vi "main004_EPICS.vi"() -> ()   [LabVIEW 2020]
uses:
  <vilib>/DAQmx/write.llb/DAQmx Write (Analog DBL 1Chan 1Samp).vi
  <vilib>/DAQmx/miscellaneous.llb/DAQmx Fill In Error Info.vi
  <vilib>/DAQmx/create/channels.llb/DAQmx Create Channel (AO-Voltage-Basic).vi
  <userlib>/caLab/Private/Put_DBL_PV.vi
  libs/Newport ESP301/Newport ESP301.lvlib
panel:
  in  "Path file to softIOC.dbd":string="C:\\Program Files (x86)\\National Instruments\\LabVIEW 2015\\user.lib\\caLab\\lib"
  out "IOC started":bool=TRUE
  in  "Config File":path=path "T:/trARPES/Labview/Front ends/METIS_delayscan/delayScanEPICS.conf" caption="Soft IOC configuration file"
  in  "Configuration Set":T1(array[cluster])=[{"PV name"="trARPES:DelayStage:t0", "description"="Delay Stage time zero Position", "data type"="ai", "number of elements (waveform only)"=1, "element size (waveform only)"="", []}, {"PV name"="trARPES:DelayStage:p1", "description"="Delay Stage range start", "data type"="ai", "number of elements (waveform only)"=1, "element size (waveform only)"="", []}, {"PV name"="trARPES:DelayStage:p2", "description"="Delay Stage range end", "data type"="ai", "number of elements (waveform only)"=1, "element size (waveform only)"="", []}, {"PV name"="trARPES:DelayStage:Pos", "description"="Current Delay Stage position", "data type"="ai", "number of elements (waveform only)"=1, "element size (waveform only)"="", []}]
  in  "Boolean":bool
  out "a":waveform(dbl)(graph)={"t0"=timestamp(3671595662.0560446 s since 1904-01-01), "dt"=1.0, "Y"=[-30.78165]}
  out "Waveform Chart":dbl(graph)=5.25341140860948
  out "x*y":dbl=-1720.2895668242609
  in  "physical channels":tag="Dev1/ao1"
  out "DAC error":errorcluster
  out "ESP error":errorcluster
  out "run?":bool
  in  "set_vel":bool
  in  "velocity [fs/s]":dbl=66.71281903963042
  in  "vel_mm":dbl=0.2 caption="velocity [mm/s]"
  out "meas. velocity":dbl
  in  "stop":bool
  out "output voltage":dbl
  in  "start":bool
  in  "go2p1":bool
  out "position [fs]":dbl=-215785.61526054132
  out "position [mm]":dbl=-30.78165
  in  "p2 [mm]":dbl=1.6200981145
  in  "p1 [mm]":dbl=1.4702018855
  in  "interpolate output":bool
  in  "t2 [fs]":dbl=375.58059249108845
  in  "t1 [fs]":dbl=-624.4194075089106
  in  "t0 [mm]":dbl=1.5638
  in  "Axis (1)":i32=3 min=1 max=3
  in  "Serial Link (RS232)":enum16{"RS232", "USB"}(ring)
  in  "VISA resource name":refnum<visa-resource-name>="COM8"
  in  "main_close":bool=TRUE
  # "Always use CLOSE button to correctly disconnect the device. STOP program afterwards."
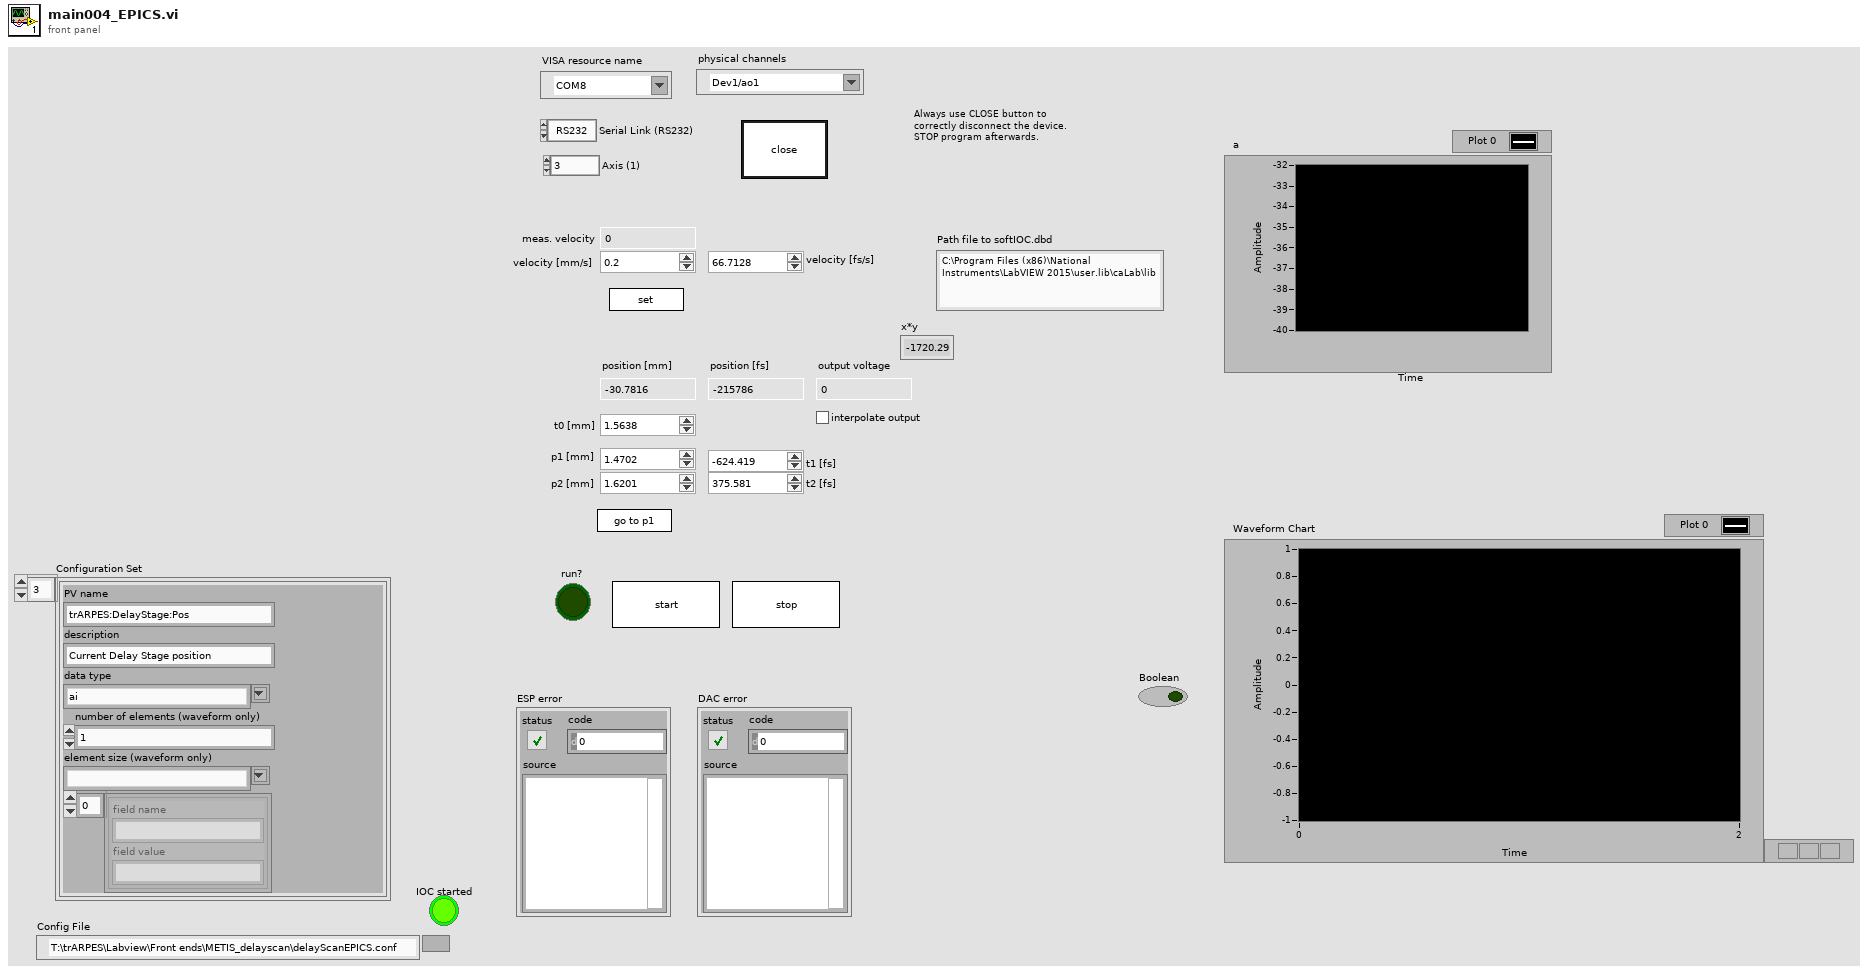
[diagram p1: front panel]
types:
  T1 = cluster{"PV name":string, "description":string, "data type":string, "number of elements (waveform only)":i32, "element size (waveform only)":string, cluster{"field name":string, "field value":string}[]}[]
  T2 = cluster{"dev1_data":refnum<queue>, "dev2_data":refnum<queue>}
  T3 = cluster{"dev1_cmd":refnum<queue>, "dev2_cmd":refnum<queue>}
  T4 = cluster{"PV Name":string, "Data Type":string, "Fields":cluster{"Field Name":string, "Field Value":string}[]}[]
  T5 = cluster{"PV Name":string, "Data Type":string, "Fields":cluster{"Field Name":string, "Field Value":string}[]}
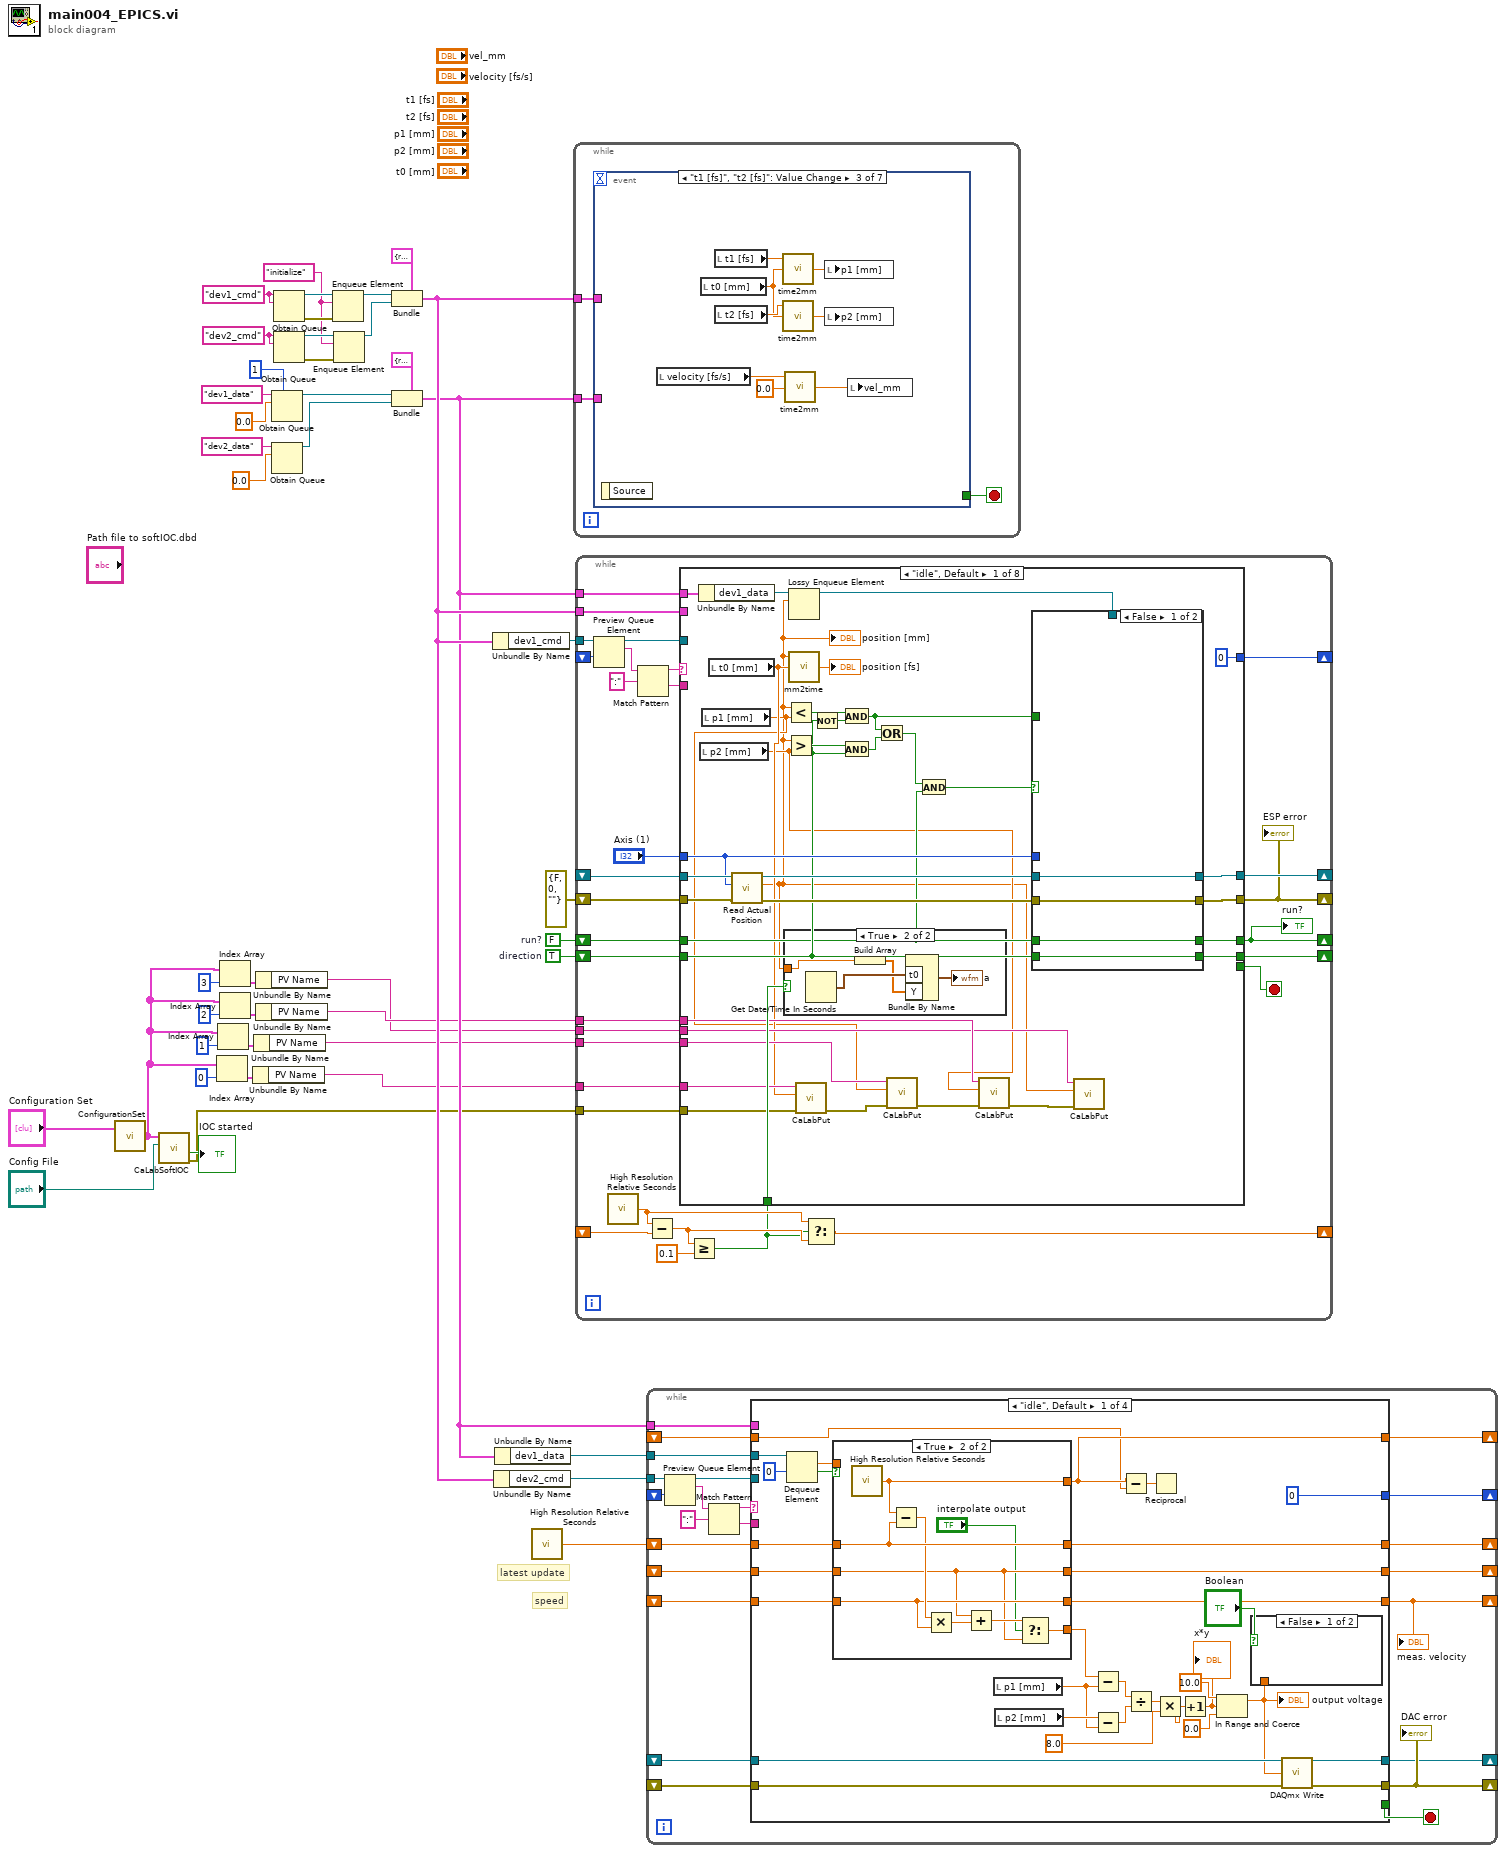
[diagram p0: block diagram]
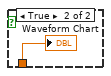
[diagram p2: hidden frame]
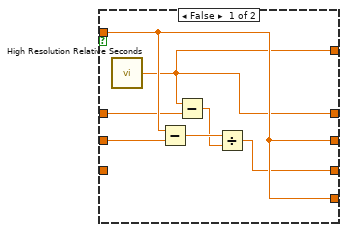
[diagram p3: hidden frame]
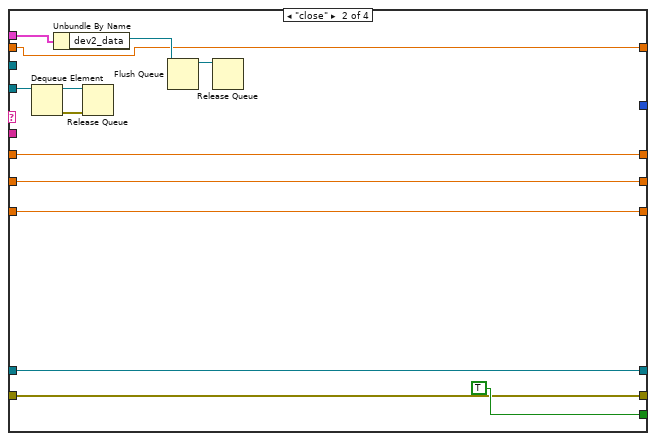
[diagram p4: hidden frame]
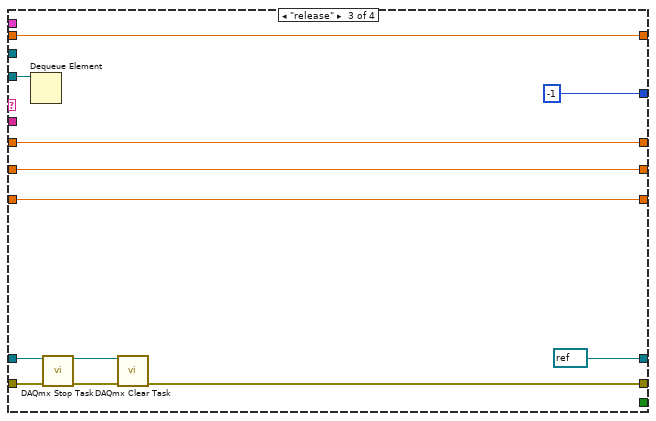
[diagram p5: hidden frame]
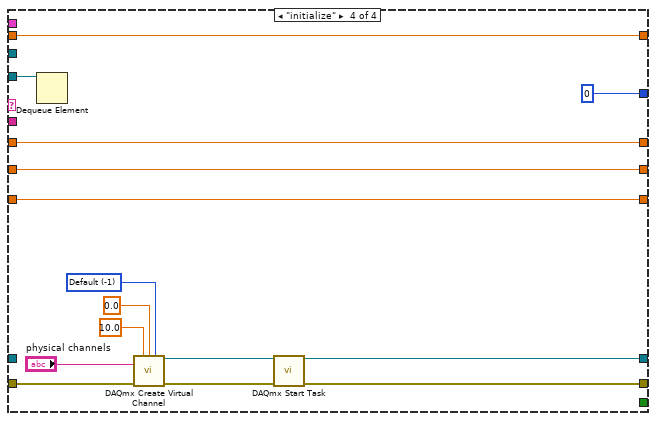
[diagram p6: hidden frame]
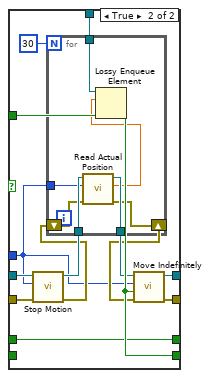
[diagram p8: hidden frame]
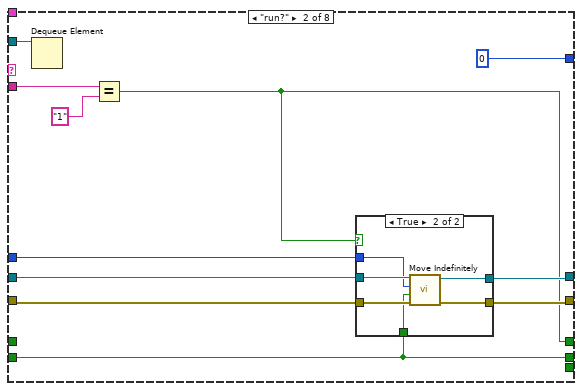
[diagram p9: hidden frame]
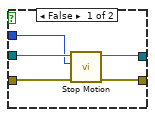
[diagram p10: hidden frame]
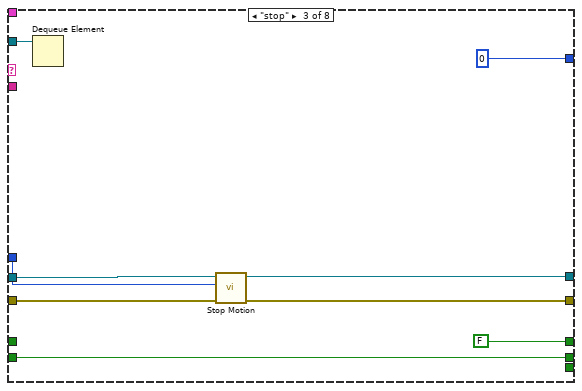
[diagram p11: hidden frame]
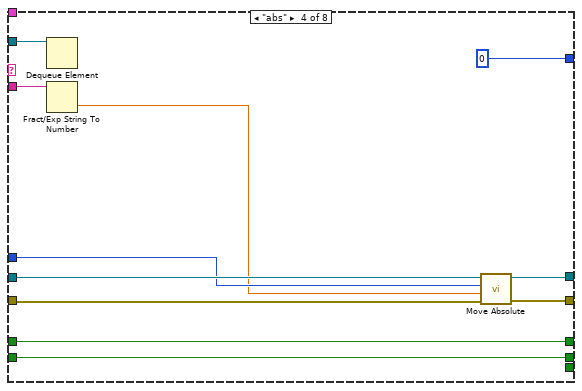
[diagram p12: hidden frame]
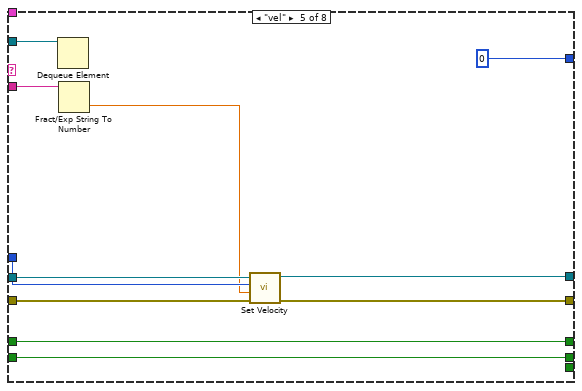
[diagram p13: hidden frame]
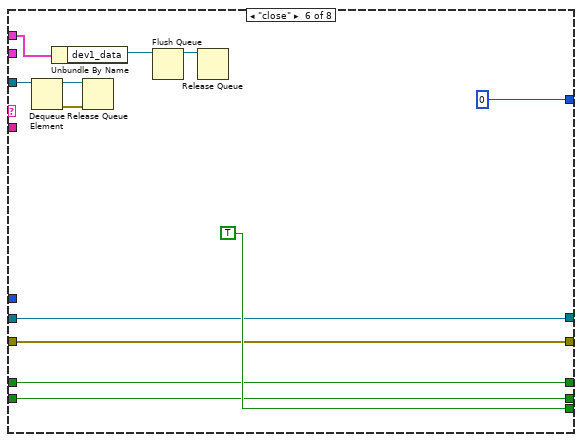
[diagram p14: hidden frame]
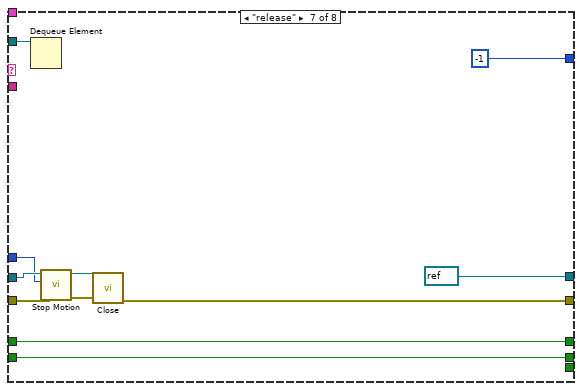
[diagram p15: hidden frame]
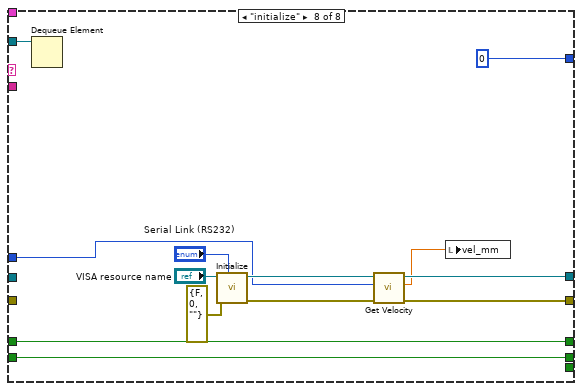
[diagram p16: hidden frame]
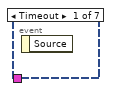
[diagram p17: hidden frame]
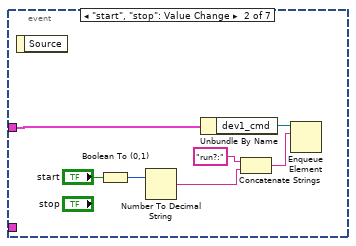
[diagram p18: hidden frame]
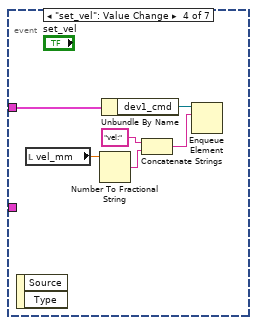
[diagram p19: hidden frame]
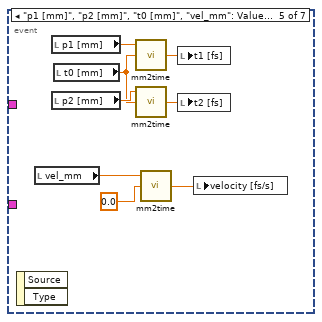
[diagram p20: hidden frame]
diagram:
  w18 = TRUE  # direction
  w21 = FALSE  # run?
  w32 = "dev2_cmd" ("name (unnamed)")
  w38 = "initialize" ("element")
  w33 = "dev1_cmd" ("name (unnamed)")
  # "speed"
  # "latest update"
  n1 = call <userlib>:"ConfigurationSet.vi"("Configuration Set"="Configuration Set") -> ("PV set"=w5:T4)  [unwired: 1 in]
  n2 = call <userlib>:"CaLabSoftIOC.vi"("Config File"="Config File", "PV set"=w5) -> ("error out"=w13:errorcluster, "IOC started"=→"IOC started":bool)  [unwired: 4 in, 2 out]
  n3 = Index Array(array=w5, index=0) -> (element=w16:T5)
  n4 = Index Array(array=w5, index=1) -> (element=w10:T5)
  n5 = Index Array(array=w5, index=3) -> (element=w6:T5)
  n6 = Index Array(array=w5, index=2) -> (element=w9:T5)
  n7 = Unbundle By Name(w16) -> ("PV Name"=w12:string)
  n8 = Unbundle By Name(w10) -> ("PV Name"=w4:string)
  n9 = Unbundle By Name(w6) -> ("PV Name"=w2:string)
  n10 = Unbundle By Name(w9) -> ("PV Name"=w3:string)
  n11 = Obtain Queue(max queue size (-1, unlimited)=1, name (unnamed)="dev1_data", element data type=0.0) -> (queue out=w29:refnum<queue>)  [unwired: 2 in, 2 out]
  n12 = Obtain Queue(name (unnamed)="dev2_data", element data type=0.0) -> (queue out=w28:refnum<queue>)  [unwired: 3 in, 2 out]
  n13 = Obtain Queue(name (unnamed)=w33, element data type=w33) -> (queue out=w44:refnum<queue>, error out=w43:errorcluster)  [unwired: 3 in, 1 out]
  n14 = Obtain Queue(name (unnamed)=w32, element data type=w32) -> (queue out=w39:refnum<queue>, error out=w40:errorcluster)  [unwired: 3 in, 1 out]
  n15 = Enqueue Element(queue=w44, element=w38, error in (no error)=w43) -> (queue out=w41:refnum<queue>)  [unwired: 1 in, 2 out]
  n16 = Enqueue Element(queue=w39, element=w38, error in (no error)=w40) -> (queue out=w37:refnum<queue>)  [unwired: 1 in, 2 out]
  n17 = Bundle(cluster=T3 {"dev1_cmd"=refnum, "dev2_cmd"=refnum}, "dev1_cmd"=w41, "dev2_cmd"=w37) -> (w25:T3)
  n18 = Bundle(cluster=T2 {"dev1_data"=refnum, "dev2_data"=refnum}, "dev1_data"=w29, "dev2_data"=w28) -> (w19:T2)
  n19 = Unbundle By Name(w25) -> ("dev1_cmd"=w34:refnum<queue>)
  n20 = Unbundle By Name(w25) -> ("dev2_cmd"=w24:refnum<queue>)
  n21 = Unbundle By Name(w19) -> ("dev1_data"=w23:refnum<queue>)
  n22 = call <vilib>:"High Resolution Relative Seconds.vi"() -> ("relative seconds"=w22:dbl)
  n23 = while {
    tunnel: w25 -> [w47]
    tunnel: w19 -> [w46]
    stop <- w45 stop-if-true
    n24 = event shown="[2] \"t1 [fs]\", \"t2 [fs]\": Value Change" {
      selector: _ -> [_ _ _ _ _ _ _]
      dyn-events: _ -> [_ _ _ _ _ _ _]
      timeout: _ -> [_ _ _ _ _ _ _]
      tunnel: w47 -> [_ w51 _ w64 _ w82 w85]
      tunnel: w46 -> [_ _ _ _ _ _ _]
      tunnel: [_ _ _ _ _ _ TRUE] -> w45
      event Timeout {
        n25 = event-data() -> ()  [unwired: 1 in, 1 out]
      }
      event "start", "stop": Value Change {
        n26 = event-data() -> ()  [unwired: 1 in, 1 out]
        n27 = Boolean To (0,1)(Boolean="start") -> (0, 1=w49:i16)
        n28 = Number To Decimal String(number=w49) -> (decimal integer string=w48:string)  [unwired: 1 in]
        n29 = Unbundle By Name(w51) -> ("dev1_cmd"=w54:refnum<queue>)
        n30 = Concatenate Strings("run?:" ("string"), w48) -> (w53:string)
        n31 = Enqueue Element(queue=w54, element=w53) -> ()  [unwired: 2 in, 3 out]
      }
      event "t1 [fs]", "t2 [fs]": Value Change {
        n32 = event-data() -> ()  [unwired: 1 in, 1 out]
        n33 = local read "velocity [fs/s]"() -> (w57:dbl)
        n34 = local read "t0 [mm]"() -> (w60:dbl)
        n35 = local read "t1 [fs]"() -> (w61:dbl)
        n36 = local read "t2 [fs]"() -> (w62:dbl)
        n37 = call "time2mm.vi"("Offset (mm)"=w60, "time"=w61) -> ("position (mm)"=w58:dbl)  [unwired: 1 in]
        n38 = call "time2mm.vi"("Offset (mm)"=w60, "time"=w62) -> ("position (mm)"=w59:dbl)  [unwired: 1 in]
        n39 = call "time2mm.vi"("Offset (mm)"=0.0, "time"=w57) -> ("position (mm)"=w55:dbl)  [unwired: 1 in]
        n40 = local write "p1 [mm]"(w58) -> ()
        n41 = local write "p2 [mm]"(w59) -> ()
        n42 = local write "vel_mm"(w55) -> ()
      }
      event "set_vel": Value Change {
        n43 = event-data() -> ()  [unwired: 1 in, 2 out]
        n44 = local read "vel_mm"() -> (w63:dbl)
        n45 = Number To Fractional String(number=w63) -> (F-format string=w67:string)  [unwired: 3 in]
        n46 = Unbundle By Name(w64) -> ("dev1_cmd"=w68:refnum<queue>)
        n47 = Concatenate Strings("vel:" ("string"), w67) -> (w66:string)
        n48 = Enqueue Element(queue=w68, element=w66) -> ()  [unwired: 2 in, 3 out]
      }
      event "p1 [mm]", "p2 [mm]", "t0 [mm]", "vel_mm": Value Change {
        n49 = event-data() -> ()  [unwired: 1 in, 2 out]
        n50 = local read "vel_mm"() -> (w71:dbl)
        n51 = local read "p1 [mm]"() -> (w75:dbl)
        n52 = local read "p2 [mm]"() -> (w76:dbl)
        n53 = local read "t0 [mm]"() -> (w74:dbl)
        n54 = call "mm2time.vi"("Offset (mm)"=w74, "distance (mm)"=w75) -> ("time in fs"=w72:dbl)  [unwired: 1 in]
        n55 = call "mm2time.vi"("Offset (mm)"=w74, "distance (mm)"=w76) -> ("time in fs"=w73:dbl)  [unwired: 1 in]
        n56 = call "mm2time.vi"("Offset (mm)"=0.0, "distance (mm)"=w71) -> ("time in fs"=w70:dbl)  [unwired: 1 in]
        n57 = local write "t1 [fs]"(w72) -> ()
        n58 = local write "t2 [fs]"(w73) -> ()
        n59 = local write "velocity [fs/s]"(w70) -> ()
      }
      event "go2p1": Value Change {
        n60 = event-data() -> ()  [unwired: 1 in, 2 out]
        n61 = local read "p1 [mm]"() -> (w77:dbl)
        n62 = Number To Fractional String(number=w77) -> (F-format string=w80:string)  [unwired: 3 in]
        n63 = Unbundle By Name(w82) -> ("dev1_cmd"=w81:refnum<queue>)
        n64 = Concatenate Strings("abs:" ("string"), w80) -> (w78:string)
        n65 = Enqueue Element(queue=w81, element=w78) -> ()  [unwired: 2 in, 3 out]
      }
      event "main_close": Value Change {
        n66 = event-data() -> ()  [unwired: 1 in, 1 out]
        n67 = Cluster To Array(cluster=w85) -> (array=w84:refnum<queue>[])
        n68 = for {
          tunnel: w84 -> [w90] mode=indexing
          n69 = Flush Queue(queue=w90) -> (queue out=w86:refnum<queue>)  [unwired: 1 in, 2 out]
          n70 = Enqueue Element(queue=w86, element="release") -> (queue out=w88:refnum<queue>)  [unwired: 2 in, 2 out]
          n71 = Enqueue Element(queue=w88, element="close") -> ()  [unwired: 2 in, 3 out]
        }
      }
    }
  }
  n72 = while {
    tunnel: w25 -> [w116]
    tunnel: w34 -> [w121]
    tunnel: w19 -> [w113]
    shift-right: [w111] -> _
    shift-left: _ -> [w112]
    shift-right: [w110] -> _
    shift-left: _ -> [w107]
    shift-right: [w109] -> _
    shift-left: errorcluster {"status"=FALSE, "code"=0, "source"=""} ("error out") -> [w108]
    shift-right: [w104] -> _
    shift-left: w21 -> [w105]
    shift-right: [w102] -> _
    shift-left: w18 -> [w103]
    shift-right: [w96] -> _
    shift-left: _ -> [w101]
    tunnel: w13 -> [w95]
    tunnel: w12 -> [w94]
    tunnel: w4 -> [w93]
    tunnel: w3 -> [w92]
    tunnel: w2 -> [w91]
    stop <- w114 stop-if-true
    n73 = Preview Queue Element(queue=w121, timeout in ms (-1)=w112) -> (queue out=w115:refnum<queue>, element=w120:string)  [unwired: 1 in, 2 out]
    n74 = call <vilib>:"High Resolution Relative Seconds.vi"() -> ("relative seconds"=w98:dbl)
    n75 = Match Pattern(string=w120, regular expression=":") -> (before substring=w118:string, after substring=w117:string)  [unwired: 1 in, 2 out]
    n76 = Subtract(x=w98, y=w101) -> (x-y=w99:dbl)
    n77 = Greater Or Equal?(x=w99, y=0.1) -> (x >= y?=w97:bool)
    n78 = case shown="\"idle\", Default" w118 {
      tunnel: w117 -> [_ w196 _ w226 w233 _ _ _]
      tunnel: w116 -> [_ _ _ _ _ _ _ _]
      tunnel: w115 -> [_ w194 w209 w227 w231 w250 w260 w270]
      tunnel: [_ _ _ _ _ TRUE _ _] -> w114
      tunnel: w113 -> [w156 _ _ _ _ w242 _ _]
      tunnel: [0 0 0 0 0 0 -1 0] -> w111
      tunnel: [w153 w191 w214 w223 w238 w246 refnum<visa-resource-name> refnum ("VISA resource name out") w266] -> w110
      tunnel: [w152 w190 w213 w222 w237 w245 w259 w265] -> w109
      tunnel: w108 -> [w148 w188 w215 w224 w236 w245 w255 _]
      tunnel: w107 -> [w150 w189 w216 w225 w235 w246 w252 _]
      tunnel: "Axis (1)" -> [w149 w192 w212 w221 w234 _ w251 w267]
      tunnel: w105 -> [w137 _ _ w218 w229 w243 w257 w271]
      tunnel: [w136 w187 FALSE ("run?") w218 w229 w243 w257 w271] -> w104
      tunnel: w103 -> [w138 w186 w208 w217 w228 w239 w256 w262]
      tunnel: [w139 w186 w208 w217 w228 w239 w256 w262] -> w102
      tunnel: w97 -> [w135 _ _ _ _ _ _ _]
      tunnel: w95 -> [w133 _ _ _ _ _ _ _]
      tunnel: w94 -> [w129 _ _ _ _ _ _ _]
      tunnel: w93 -> [w128 _ _ _ _ _ _ _]
      tunnel: w92 -> [w127 _ _ _ _ _ _ _]
      tunnel: w91 -> [w126 _ _ _ _ _ _ _]
      frame "idle", Default {
        n79 = Unbundle By Name(w156) -> ("dev1_data"=w155:refnum<queue>)
        n80 = local read "p2 [mm]"() -> (w123:dbl)
        n81 = local read "p1 [mm]"() -> (w124:dbl)
        n82 = local read "t0 [mm]"() -> (w125:dbl)
        n83 = call "Read Actual Position.vi"("error in (no error)"=w148, "Axis (1)"=w149, "VISA resource name"=w150) -> ("error out"=w147:errorcluster, "Position (units)"=w122:dbl, "VISA resource name out"=w146:refnum<visa-resource-name>)  [unwired: 2 in]
        "position [mm]" <- w122
        n84 = case shown="True" w135 {
          tunnel: w122 -> [_ w161]
          frame False {
          }
          frame True {
            n85 = Get Date/Time In Seconds() -> (seconds since 1Jan1904=w160:timestamp)
            n86 = Build Array(w161) -> (w159:dbl[])
            n87 = Bundle By Name("t0"=w160, "Y"=w159) -> (→"a":waveform(dbl))  [unwired: 1 in]
          }
        }
        n88 = Less?(x=w122, y=w124) -> (x < y?=w144:bool)
        n89 = Greater?(x=w122, y=w123) -> (0:w143:bool)
        n90 = Lossy Enqueue Element(queue=w155, element=w122) -> (queue out=w134:refnum<queue>)  [unwired: 1 in, 3 out]
        n91 = call "mm2time.vi"("Offset (mm)"=w125, "distance (mm)"=w122) -> ("time in fs"=→"position [fs]":dbl)  [unwired: 1 in]
        n92 = call-poly <userlib>:"CaLabPut.vi"("Error in (no error)"=w133, "Value"=w125, "PV Name"=w129) -> ("Error out"=w132:errorcluster)  [unwired: 5 in, 3 out]
        n93 = Not(x=w138) -> (.not. x?=w145:bool)
        n94 = And(x=w144, y=w145) -> (x .and. y?=w140:bool)
        n95 = And(x=w143, y=w138) -> (x .and. y?=w142:bool)
        n96 = Or(x=w140, y=w142) -> (x .or. y?=w141:bool)
        n97 = call-poly <userlib>:"CaLabPut.vi"("Error in (no error)"=w132, "Value"=w124, "PV Name"=w128) -> ("Error out"=w131:errorcluster)  [unwired: 5 in, 3 out]
        n98 = And(x=w141, y=w137) -> (x .and. y?=w151:bool)
        n99 = call-poly <userlib>:"CaLabPut.vi"("Error in (no error)"=w131, "Value"=w123, "PV Name"=w127) -> ("Error out"=w130:errorcluster)  [unwired: 5 in, 3 out]
        n100 = case shown="False" w151 {
          tunnel: w146 -> [w165 w176]
          tunnel: w147 -> [w164 w175]
          tunnel: [w165 w178] -> w153
          tunnel: [w164 w177] -> w152
          tunnel: w149 -> [_ w168]
          tunnel: w140 -> [_ w174]
          tunnel: [w163 w174] -> w139
          tunnel: w138 -> [w163 _]
          tunnel: w137 -> [w162 w173]
          tunnel: [w162 w173] -> w136
          tunnel: w134 -> [_ w167]
          frame False {
          }
          frame True {
            n101 = call "Stop Motion.vi"("error in (no error)"=w175, "Axis (1)"=w168, "VISA resource name"=w176) -> ("error out"=w170:errorcluster, "VISA resource name out"=w172:refnum<visa-resource-name>)  [unwired: 3 in]
            n102 = for {
              N: 30 -> [_]
              tunnel: w172 -> [w185]
              tunnel: [w184] -> w171
              shift-right: [w182] -> w169
              shift-left: w170 -> [w183]
              tunnel: w168 -> [w181]
              tunnel: w167 -> [w180]
              n103 = call "Read Actual Position.vi"("error in (no error)"=w183, "Axis (1)"=w181, "VISA resource name"=w185) -> ("error out"=w182:errorcluster, "Position (units)"=w179:dbl, "VISA resource name out"=w184:refnum<visa-resource-name>)  [unwired: 2 in]
              n104 = Lossy Enqueue Element(queue=w180, element=w179) -> ()  [unwired: 1 in, 4 out]
            }
            n105 = call "Move Indefinitely.vi"("error in (no error)"=w169, "Move Direction (+)"=w174, "Axis (1)"=w168, "VISA resource name"=w171) -> ("error out"=w177:errorcluster, "VISA resource name out"=w178:refnum<visa-resource-name>)  [unwired: 2 in]
          }
        }
        n106 = call-poly <userlib>:"CaLabPut.vi"("Error in (no error)"=w130, "Value"=w122, "PV Name"=w126) -> ()  [unwired: 5 in, 4 out]
      }
      frame "run?" {
        n107 = Dequeue Element(queue=w194) -> ()  [unwired: 2 in, 4 out]
        n108 = Equal?(x=w196, y="1") -> (x = y?=w187:bool)
        n109 = case shown="True" w187 {
          tunnel: w189 -> [w201 w207]
          tunnel: w188 -> [w198 w206]
          tunnel: w192 -> [w197 w205]
          tunnel: [w200 w204] -> w191
          tunnel: [w199 w203] -> w190
          tunnel: w186 -> [_ w202]
          frame False {
            n110 = call "Stop Motion.vi"("error in (no error)"=w198, "Axis (1)"=w197, "VISA resource name"=w201) -> ("error out"=w199:errorcluster, "VISA resource name out"=w200:refnum<visa-resource-name>)  [unwired: 3 in]
          }
          frame True {
            n111 = call "Move Indefinitely.vi"("error in (no error)"=w206, "Move Direction (+)"=w202, "Axis (1)"=w205, "VISA resource name"=w207) -> ("error out"=w203:errorcluster, "VISA resource name out"=w204:refnum<visa-resource-name>)  [unwired: 2 in]
          }
        }
      }
      frame "stop" {
        n112 = Dequeue Element(queue=w209) -> ()  [unwired: 2 in, 4 out]
        n113 = call "Stop Motion.vi"("error in (no error)"=w215, "Axis (1)"=w212, "VISA resource name"=w216) -> ("error out"=w213:errorcluster, "VISA resource name out"=w214:refnum<visa-resource-name>)  [unwired: 3 in]
      }
      frame "abs" {
        n114 = Dequeue Element(queue=w227) -> ()  [unwired: 2 in, 4 out]
        n115 = Fract/Exp String To Number(string=w226) -> (number=w220:dbl)  [unwired: 3 in, 1 out]
        n116 = call "Move Absolute.vi"("error in (no error)"=w224, "Position (0 units)"=w220, "Axis (1)"=w221, "VISA resource name"=w225) -> ("error out"=w222:errorcluster, "VISA resource name out"=w223:refnum<visa-resource-name>)  [unwired: 2 in]
      }
      frame "vel" {
        n117 = Dequeue Element(queue=w231) -> ()  [unwired: 2 in, 4 out]
        n118 = Fract/Exp String To Number(string=w233) -> (number=w232:dbl)  [unwired: 3 in, 1 out]
        n119 = call "Set Velocity.vi"("error in (no error)"=w236, "Velocity (units/s)"=w232, "Axis (1)"=w234, "VISA resource name"=w235) -> ("error out"=w237:errorcluster, "VISA resource name out"=w238:refnum<visa-resource-name>)  [unwired: 2 in]
      }
      frame "close" {
        n120 = Dequeue Element(queue=w250) -> (queue out=w249:refnum<queue>, error out=w248:errorcluster)  [unwired: 2 in, 2 out]
        n121 = Unbundle By Name(w242) -> ("dev1_data"=w240:refnum<queue>)
        n122 = Release Queue(queue=w249, error in (no error)=w248) -> ()  [unwired: 1 in, 3 out]
        n123 = Flush Queue(queue=w240) -> (queue out=w241:refnum<queue>)  [unwired: 1 in, 2 out]
        n124 = Release Queue(queue=w241) -> ()  [unwired: 2 in, 3 out]
      }
      frame "release" {
        n125 = Dequeue Element(queue=w260) -> ()  [unwired: 2 in, 4 out]
        n126 = call "Stop Motion.vi"("error in (no error)"=w255, "Axis (1)"=w251, "VISA resource name"=w252) -> ("error out"=w254:errorcluster, "VISA resource name out"=w253:refnum<visa-resource-name>)  [unwired: 3 in]
        n127 = call "Close.vi"("error in (no error)"=w254, "VISA resource name"=w253) -> ("error out"=w259:errorcluster)  [unwired: 9 in]
      }
      frame "initialize" {
        n128 = Dequeue Element(queue=w270) -> ()  [unwired: 2 in, 4 out]
        n129 = call "Initialize.vi"("VISA resource name"="VISA resource name", "error in (no error)"=errorcluster {"status"=FALSE, "code"=0, "source"=""}, "Serial Link (RS232)"="Serial Link (RS232)") -> ("VISA resource name out"=w269:refnum<visa-resource-name>, "error out"=w268:errorcluster)  [unwired: 6 in]
        n130 = call "Get Velocity.vi"("error in (no error)"=w268, "Axis (1)"=w267, "VISA resource name"=w269) -> ("error out"=w265:errorcluster, "Velocity (units/s)"=w264:dbl, "VISA resource name out"=w266:refnum<visa-resource-name>)  [unwired: 2 in]
        n131 = local write "vel_mm"(w264) -> ()
      }
    }
    "run?" <- w104
    "ESP error" <- w109
    n132 = Select(t=w98, s=w97, f=w99) -> (s? t:f=w96:dbl)
  }
  n133 = while {
    shift-right: [w290] -> _
    shift-left: _ -> [w291]
    shift-right: [w289] -> _
    shift-left: _ -> [w288]
    tunnel: w24 -> [w287]
    shift-right: [w286] -> _
    shift-left: _ -> [w285]
    tunnel: w23 -> [w284]
    shift-right: [w283] -> _
    shift-left: _ -> [w280]
    shift-right: [w282] -> _
    shift-left: w22 -> [w281]
    shift-right: [w275] -> _
    shift-left: _ -> [w279]
    tunnel: w19 -> [w278]
    shift-right: [w277] -> _
    shift-left: _ -> [w276]
    stop <- w292 stop-if-true
    n134 = Preview Queue Element(queue=w287, timeout in ms (-1)=w291) -> (queue out=w293:refnum<queue>, element=w297:string)  [unwired: 1 in, 2 out]
    n135 = Match Pattern(string=w297, regular expression=":") -> (before substring=w295:string, after substring=w294:string)  [unwired: 1 in, 2 out]
    n136 = case shown="\"idle\", Default" w295 {
      tunnel: w294 -> [_ _ _ _]
      tunnel: w293 -> [_ w358 w369 w377]
      tunnel: [_ TRUE _ _] -> w292
      tunnel: [0 _ -1 0] -> w290
      tunnel: [w324 w354 w368 w378] -> w289
      tunnel: w288 -> [w322 w354 w365 w385]
      tunnel: [w325 w353 refnum<k21> refnum ("task out") w379] -> w286
      tunnel: w285 -> [w323 w353 w366 _]
      tunnel: w284 -> [w326 _ _ _]
      tunnel: [w320 w351 w361 w374] -> w283
      tunnel: [w319 w352 w362 w375] -> w282
      tunnel: w281 -> [w317 w352 w362 w375]
      tunnel: w280 -> [w318 w351 w361 w374]
      tunnel: [w316 w350 w360 w373] -> w275
      tunnel: w279 -> [w315 w350 w360 w373]
      tunnel: w278 -> [_ w347 _ _]
      tunnel: [w304 w346 w359 w371] -> w277
      tunnel: w276 -> [w303 w346 w359 w371]
      frame "idle", Default {
        n137 = Dequeue Element(queue=w326, timeout in ms (-1)=0) -> (element=w321:dbl, timed out?=w305:bool)  [unwired: 1 in, 2 out]
        n138 = case shown="True" w305 {
          tunnel: w321 -> [w336 _]
          tunnel: [w336 w338] -> w314
          tunnel: [w336 w340] -> w320
          tunnel: [w330 w345] -> w319
          tunnel: w318 -> [w335 w340]
          tunnel: w317 -> [w334 w345]
          tunnel: [w331 w342] -> w316
          tunnel: w315 -> [_ w342]
          tunnel: [w330 w337] -> w304
          frame False {
            n139 = call <vilib>:"High Resolution Relative Seconds.vi"() -> ("relative seconds"=w330:dbl)
            n140 = Subtract(x=w336, y=w335) -> (x-y=w333:dbl)
            n141 = Subtract(x=w330, y=w334) -> (x-y=w332:dbl)
            n142 = Divide(x=w333, y=w332) -> (x/y=w331:dbl)
          }
          frame True {
            n143 = call <vilib>:"High Resolution Relative Seconds.vi"() -> ("relative seconds"=w337:dbl)
            n144 = Subtract(x=w337, y=w345) -> (x-y=w344:dbl)
            n145 = Multiply(x=w344, y=w342) -> (x*y=w343:dbl)
            n146 = Add(x=w340, y=w343) -> (x+y=w341:dbl)
            n147 = Select(t=w341, s="interpolate output", f=w340) -> (s? t:f=w338:dbl)
          }
        }
        n148 = local read "p1 [mm]"() -> (w312:dbl)
        n149 = local read "p2 [mm]"() -> (w313:dbl)
        n150 = Subtract(x=w314, y=w312) -> (x-y=w311:dbl)
        n151 = Subtract(x=w313, y=w312) -> (x-y=w310:dbl)
        n152 = Subtract(x=w304, y=w303) -> (x-y=w302:dbl)
        n153 = Divide(x=w311, y=w310) -> (x/y=w309:dbl)
        n154 = Reciprocal(x=w302) -> ()  [unwired: 1 out]
        n155 = Multiply(x=w309, y=8.0) -> (x*y=w300:dbl)
        n156 = Increment(x=w300) -> (x+1=w299:dbl)
        "x*y" <- w299
        n157 = In Range and Coerce(upper limit=10.0, x=w299, lower limit=0.0) -> (coerced(x)=w301:dbl)  [unwired: 1 out]
        "output voltage" <- w301
        n158 = case shown="False" "Boolean" {
          tunnel: w301 -> [_ w329]
          frame False {
          }
          frame True {
            "Waveform Chart" <- w329
          }
        }
        n159 = call-poly <vilib>:"DAQmx Write.vi"("task/channels in"=w323, "data"=w301, "error in"=w322) -> ("task out"=w325:refnum<k21>, "error out"=w324:errorcluster)  [unwired: 10 in, 1 out]
      }
      frame "close" {
        n160 = Dequeue Element(queue=w358) -> (queue out=w357:refnum<queue>, error out=w356:errorcluster)  [unwired: 2 in, 2 out]
        n161 = Unbundle By Name(w347) -> ("dev2_data"=w348:refnum<queue>)
        n162 = Release Queue(queue=w357, error in (no error)=w356) -> ()  [unwired: 1 in, 3 out]
        n163 = Flush Queue(queue=w348) -> (queue out=w349:refnum<queue>)  [unwired: 1 in, 2 out]
        n164 = Release Queue(queue=w349) -> ()  [unwired: 2 in, 3 out]
      }
      frame "release" {
        n165 = Dequeue Element(queue=w369) -> ()  [unwired: 2 in, 4 out]
        n166 = call <vilib>:"DAQmx Stop Task.vi"("task/channels in"=w366, "error in"=w365) -> ("task out"=w364:refnum<k21>, "error out"=w363:errorcluster)  [unwired: 12 in]
        n167 = call <vilib>:"DAQmx Clear Task.vi"("task in"=w364, "error in"=w363) -> ("error out"=w368:errorcluster)  [unwired: 13 in]
      }
      frame "initialize" {
        w382 = -1 items=["Default"=-1, "RSE"=10083, "Differential"=10106, "Pseudodifferential"=12529] ("output terminal configuration")
        n168 = Dequeue Element(queue=w377) -> ()  [unwired: 2 in, 4 out]
        n169 = call-poly <vilib>:"DAQmx Create Virtual Channel.vi"("maximum value"=10.0, "minimum value"=0.0, "output terminal configuration"=w382, "physical channels"="physical channels", "error in"=w385) -> ("task out"=w381:refnum<k21>, "error out"=w380:errorcluster)  [unwired: 9 in]
        n170 = call <vilib>:"DAQmx Start Task.vi"("task/channels in"=w381, "error in"=w380) -> ("task out"=w379:refnum<k21>, "error out"=w378:errorcluster)  [unwired: 12 in]
      }
    }
    "meas. velocity" <- w275
    "DAC error" <- w289
  }
